vi "UnCompress Image (DBDE) (SubVI).vi"(0 "Data Array":u8[](array[numeric]), 2 "Bit Depth Array":u8[](array[numeric]), 4 "Min. Array":u8[](array[numeric]), 8 "Block Size":i32, 10 "Image Width":i32, 12 "Image Height":i32) -> (14 "Image Array Out":u8[][](array[numeric]))   [LabVIEW 2015]
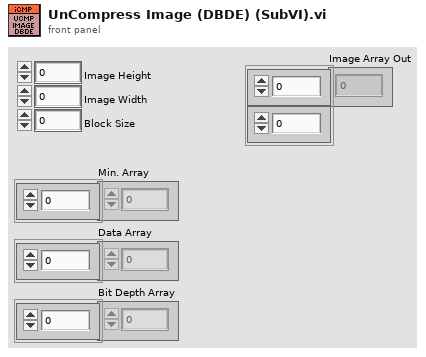
[diagram p1: front panel]
types:
  T1 = enum16{"big-endian, network order", "native, host order", "little-endian"}
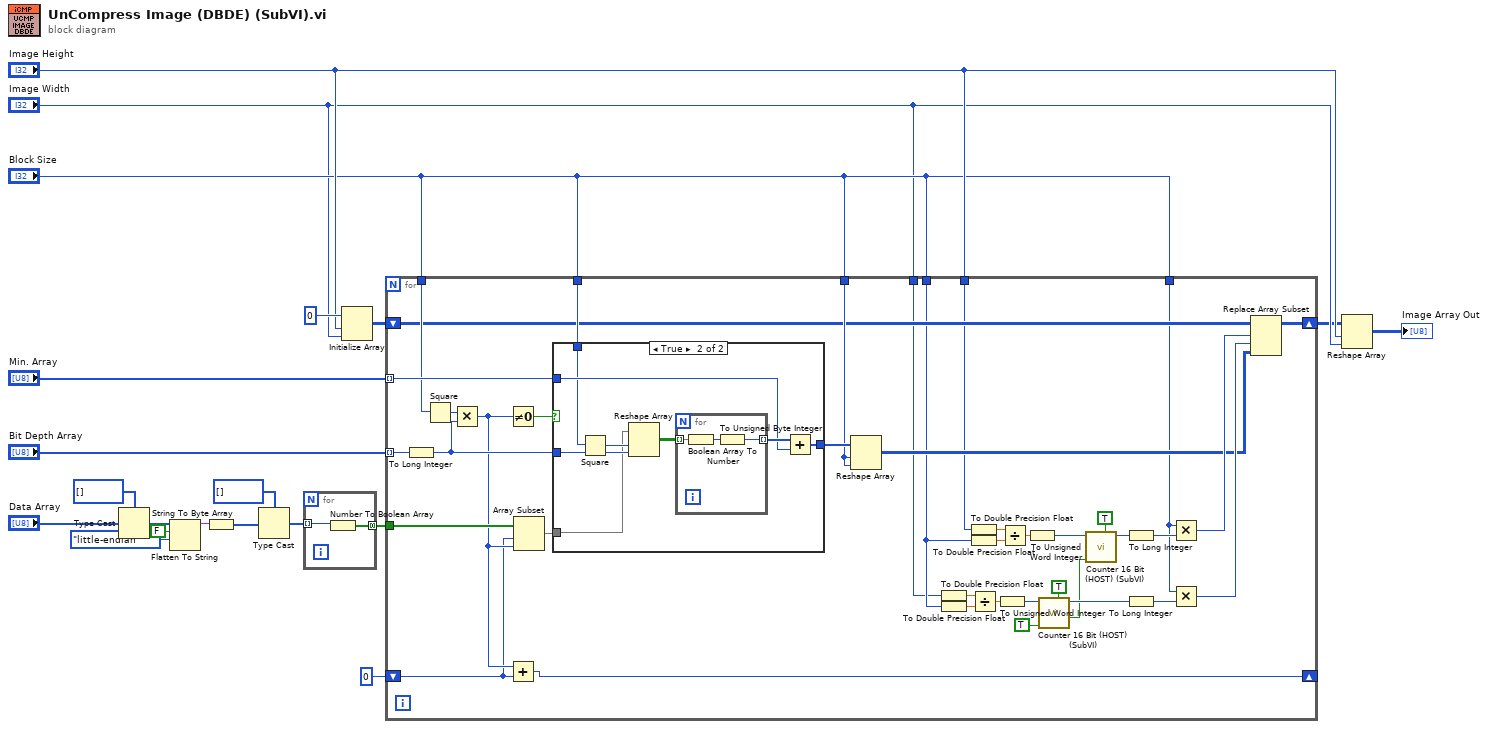
[diagram p0: block diagram]
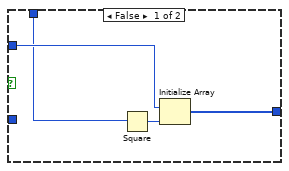
[diagram p2: hidden frame]
diagram:
  n1 = Type Cast(type=u64[] [] ("Boolean array"), x="Data Array") -> (*(type *) &x=w12:u64[])
  n2 = Flatten To String(anything=w12, prepend array or string size? (T)=FALSE, byte order (0:big-endian, network order)=T1."little-endian") -> (data string=w9:string)  [unwired: 1 in, 2 out]
  n3 = String To Byte Array(string=w9) -> (unsigned byte array=w7:u8[])
  n4 = Type Cast(type=u64[] [] ("Boolean array"), x=w7) -> (*(type *) &x=w6:u64[])
  n5 = for {
    tunnel: w6 -> [w22] mode=indexing
    tunnel: [w21] -> w13 mode=concatenating
    n6 = Number To Boolean Array(number=w22) -> (Boolean array=w21:bool[])
  }
  n7 = Initialize Array(u8 0 ("element"), "Image Height", "Image Width") -> (w5:u8[][])
  n8 = for {
    tunnel: "Min. Array" -> [w59] mode=indexing
    tunnel: "Bit Depth Array" -> [w58] mode=indexing
    shift-right: [w61] -> _
    shift-left: 0 ("y") -> [w48]
    tunnel: "Block Size" -> [w55]
    tunnel: "Block Size" -> [w56]
    tunnel: "Block Size" -> [w52]
    tunnel: w13 -> [w51]
    shift-right: [w29] -> w1
    shift-left: w5 -> [w28]
    tunnel: "Block Size" -> [w26]
    tunnel: "Image Height" -> [w25]
    tunnel: "Block Size" -> [w24]
    tunnel: "Image Width" -> [w23]
    n9 = To Long Integer(number=w58) -> (32bit integer=w53:i32)
    n10 = Square(x=w55) -> (x^2=w54:i32)
    n11 = Multiply(x=w54, y=w53) -> (x*y=w49:i32)
    n12 = Not Equal To 0?(x=w49) -> (x != 0?=w57:bool)
    n13 = Add(x=w49, y=w48) -> (x+y=w61:i32)
    n14 = Array Subset(array=w51, index=w48, length=w49) -> (w50:bool[])
    n15 = case shown="True" w57 {
      tunnel: [w64 w72] -> w60
      tunnel: w59 -> [w65 w71]
      tunnel: w53 -> [_ w70]
      tunnel: w52 -> [w63 w68]
      tunnel: w50 -> [_ w67]
      frame False {
        n16 = Square(x=w63) -> (x^2=w62:i32)
        n17 = Initialize Array(w65, w62) -> (w64:u8[])
      }
      frame True {
        n18 = Square(x=w68) -> (x^2=w69:i32)
        n19 = Reshape Array(w67, w69, w70) -> (w66:bool[][])
        n20 = for {
          tunnel: w66 -> [w76] mode=indexing
          tunnel: [w74] -> w73 mode=indexing
          n21 = Boolean Array To Number(Boolean array=w76) -> (number=w75:u32)
          n22 = To Unsigned Byte Integer(number=w75) -> (unsigned 8bit integer=w74:u8)
        }
        n23 = Add(x=w73, y=w71) -> (x+y=w72:u8[])
      }
    }
    n24 = Reshape Array(w60, w56, w56) -> (w27:u8[][])
    n25 = To Double Precision Float(number=w23) -> (double precision float=w40:dbl)
    n26 = To Double Precision Float(number=w24) -> (double precision float=w39:dbl)
    n27 = To Double Precision Float(number=w25) -> (double precision float=w42:dbl)
    n28 = To Double Precision Float(number=w24) -> (double precision float=w43:dbl)
    n29 = Divide(x=w40, y=w39) -> (x/y=w38:dbl)
    n30 = To Unsigned Word Integer(number=w38) -> (unsigned 16bit integer=w41:u16)
    n31 = Divide(x=w42, y=w43) -> (x/y=w44:dbl)
    n32 = To Unsigned Word Integer(number=w44) -> (unsigned 16bit integer=w45:u16)
    n33 = call "Counter 16 Bit (HOST) (SubVI).vi"("Auto RESET"=TRUE, "Enable"=TRUE, "Max. Count"=w41) -> ("Count End?"=w30:bool, "Count"=w32:u16)  [unwired: 6 in, 1 out]
    n34 = call "Counter 16 Bit (HOST) (SubVI).vi"("Auto RESET"=TRUE, "Enable"=w30, "Max. Count"=w45) -> ("Count"=w33:u16)  [unwired: 6 in, 2 out]
    n35 = To Long Integer(number=w33) -> (32bit integer=w36:i32)
    n36 = To Long Integer(number=w32) -> (32bit integer=w37:i32)
    n37 = Multiply(x=w26, y=w36) -> (x*y=w34:i32)
    n38 = Multiply(x=w26, y=w37) -> (x*y=w35:i32)
    n39 = Replace Array Subset(array=w28, new element=w27, index (row)=w34, index (col)=w35) -> (w29:u8[][])
  }
  n40 = Reshape Array(w1, "Image Height", "Image Width") -> (→"Image Array Out":u8[][])
